vi "FTW-CSV-Variant-Serialize.vi"(0 "Variant":variant, 9 "String Quotes":bool, 11 "error in":errorcluster, 12 "Real Format":string="%#_15g", 13 "Timestamp Format":string="%^<%Y-%m-%dT%H:%M:%S%3uZ>T", 14 "Line Ending":string="\n") -> (4 "CSV String":string, 15 "error out":errorcluster)   [LabVIEW 2015]
uses:
  FTW-CSV-SerializeOptions.ctl
  <vilib>/Utility/Data Type/NI_Data Type.lvlib
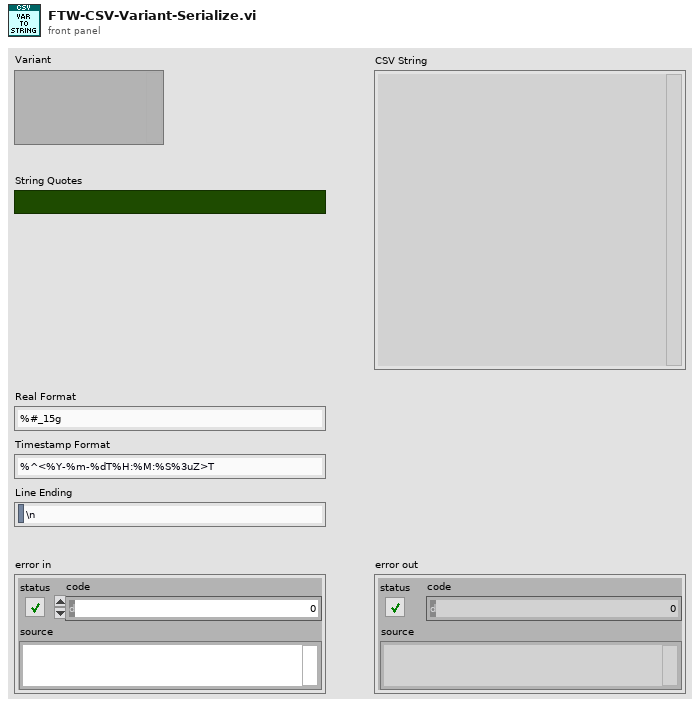
[diagram p1: front panel]
types:
  T1 = typedef "FTW-CSV-SerializeOptions.ctl" = cluster{"String Quotes":bool, "Real Format":string, "Timestamp Format":string}
  T2 = typedef "NI_Data Type.lvlib/Data Type.ctl" = enum8{"Invalid Type", "Void", "I8", "I16", "I32", "I64", "U8", "U16", "U32", "U64", "Single Float", "Double Float", "Extended Float", "Single Complex", "Double Complex", "Extended Complex", "Enum U8", "Enum U16", "Enum U32", "Enum U64", "Single Float With Unit", "Double Float With Unit", "Extended Float With Unit", "Single Complex with Unit", "Double Complex with Unit", "Extended Complex with Unit", "Boolean", "String", "Path", "Picture", "Tag", "Array", "Cluster", "Variant", "LV Variant", "Waveform", "Timestamp", "Digital Waveform", "Digital Data", "ExpressData", "Refnum", "External Data", "VI", "Poly VI", "LabVIEW Class Instance", "Fixed Point"}
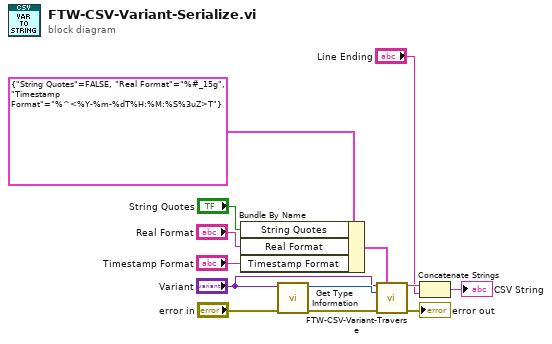
[diagram p0: block diagram]
diagram:
  n1 = Bundle By Name(cluster=T1 {"String Quotes"=FALSE, "Real Format"="%#_15g", "Timestamp Format"="%^<%Y-%m-%dT%H:%M:%S%3uZ>T"} ("Options"), "String Quotes"="String Quotes", "Real Format"="Real Format", "Timestamp Format"="Timestamp Format") -> (w10:T1)
  n2 = call <vilib>:"Get Type Information.vi"("error in (no error)"="error in", "Variant"="Variant") -> ("error out"=w8:errorcluster, "Type"=w7:T2)  [unwired: 5 in, 3 out]
  n3 = call "FTW-CSV-Variant-Traverse.vi"("Variant"="Variant", "Options"=w10, "Type"=w7, "error in"=w8) -> ("CSV String"=w11:string, "error out"=→"error out":errorcluster)  [unwired: 10 in]
  n4 = Concatenate Strings(w11, "Line Ending") -> (→"CSV String":string)
